vi "参数设置页.vi"() -> ()   [LabVIEW 2016, in "斯坦道氟化物.lvlib"]
uses:
  <vilib>/Plasmionique/MB Master/MB_Master/MB_Master.lvclass
  <vilib>/ptbypt/NI_PtbyPt.lvlib
panel:
  out "连接状态":bool
  in  "标样核查自动补测":bool caption="通讯连接"
  in  "跨度核查自动补测":bool caption="通讯连接"
  in  "零点核查自动补测":bool caption="通讯连接"
  in  "标样核查标液偏差":dbl caption="标样核查标液偏差："
  in  "跨度核查标液偏差":dbl caption="跨度核查标液偏差："
  in  "零点核查标液偏差":dbl caption="零点核查标液偏差："
  out "低量程上限":dbl caption="低量程上限："
  in  "简易流程路径":path=path "data/流程.xml"
  out "数据刷新时间":string
  in  "通讯连接":bool=TRUE
  out "MB table":enum32{"Serial", "TCP"}(tab)
  in  "请选择串口:":refnum<visa-resource-name>
  in  "IP":string="127.0.0.1"
  in  "PORT":string="1001"
  in  "通信方式选择":enum16{"串口", "TCP"}(ring)
  in  "盐度自动补偿：":bool
  out "盐度补偿值":dbl caption="盐度补偿值："
  in  "刷新":bool
  in  "测量模式":T1(ring)
  in  "参数下拉列表":u16(ring)
  in  "量程下拉列表":enum16{"低量程", "高量程"}(ring)
  in  "测试流程路径":path=path "data/流程.xml"
  in  "标样核查量程模式":T2 caption="标样核查："
  in  "加标回收量程模式":T2 caption="加标回收："
  in  "跨度核查量程模式":T2 caption="跨度核查："
  in  "零点核查量程模式":T2 caption="零点核查："
  in  "水样测试量程模式":T2 caption="水样测试："
  out "稀释度":dbl caption="稀释度："
  out "阈值（高->低）":dbl caption="阈值（高->低）："
  out "阈值（低->高）":dbl caption="阈值（低->高）："
  out "量程下限":dbl caption="量程下限："
  out "高量程上限":dbl caption="高量程上限："
  out "检出限":dbl caption="检出限："
  out "曲线截距":dbl caption="曲线截距：" format="%#.6f"
  out "曲线斜率":dbl caption="曲线斜率：" format="%#.6f"
  out "二次多项式系数":dbl caption="二次多项式系数：" format="%#.6f"
  out "消解时长":dbl caption="消解时长："
  out "消解温度":dbl caption="消解温度："
  out "测量精度":u16 caption="测量精度："
  in  "标样核查标液浓度":dbl caption="标样核查标液浓度："
  in  "跨度核查标液浓度":dbl caption="跨度核查标液浓度："
  in  "零点核查标液浓度":dbl caption="零点核查标液浓度："
  in  "跨度值":dbl caption="跨度值："
  # "日质控设置"
  # "关键参数"
  # "连接设置"
  # "mg/L"
  # "mg/L"
  # "mg/L"
  # "mg/L"
  # "±"
  # "%"
  # "%"
  # "流程设置"
  # "自动测试量程设置"
  # "mg/L"
  # "ppt"
  # "mg/L"
  # "mg/L"
  # "mg/L"
  # "mg/L"
  # "mg/L"
  # "min"
  # "℃"
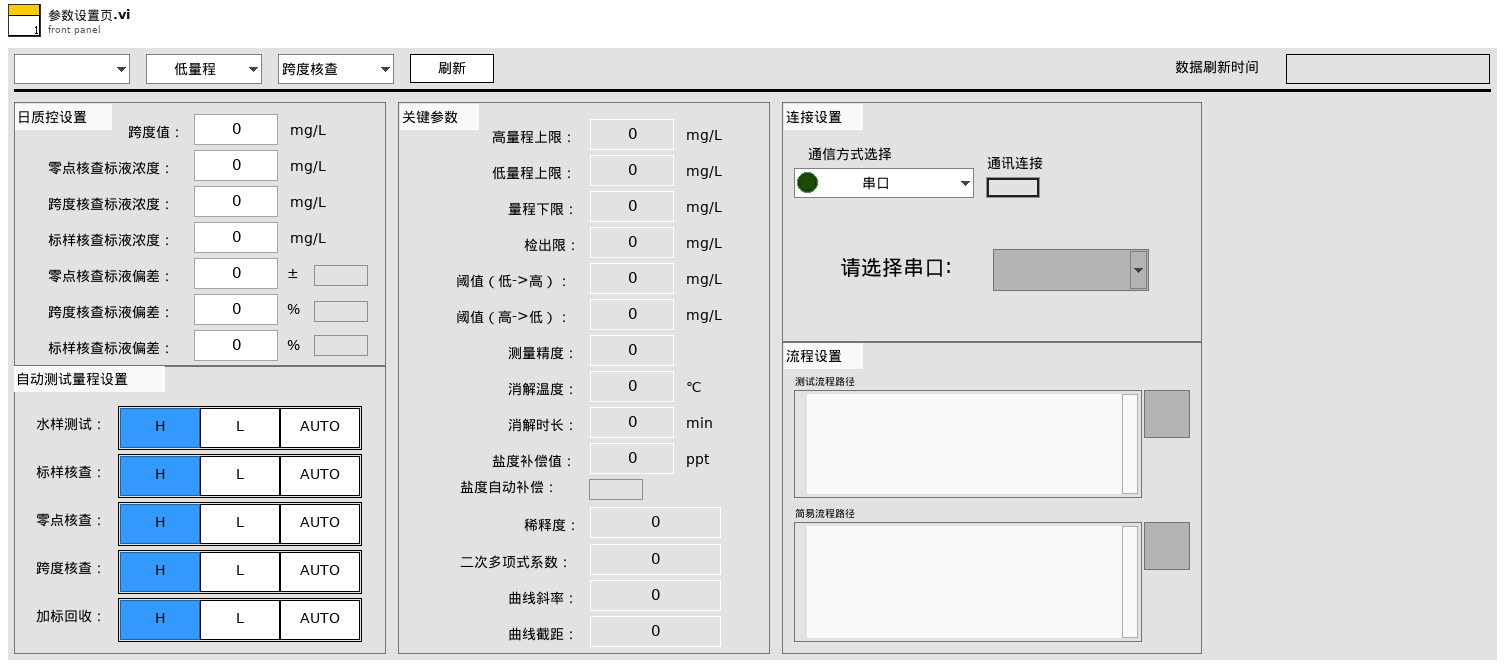
[diagram p1: front panel]
types:
  T1 = enum16{"跨度核查", "水样测量", "零点核查", "标样核查", "加标回收", "快捷测试", "空白校准", "标样校准"}
  T2 = typedef "斯坦道氟化物.lvlib/量程模式.ctl" = enum32{"H", "L", "AUTO"}
  T3 = typedef "LVStringsAndValuesArrayTypeDef_U16.ctl" = cluster{"String":string, "Value":u16}[]
  T4 = cluster{"系统时间":timestamp, "工作状态":u16, "测量模式":enum16{"待机", "连续模式", "周期模式", "定点模式", "受控模式", "手动模式"}, "告警代码":u16, "故障代码":u16, "日志代码":u16, "软件版本":u16, "F0":sgl, "F1":sgl, "F2":sgl, "F3":sgl, "T":sgl, "H":sgl, "id":u16, "flowid":u16, "量程":u16, "总磷控温温度1":sgl, "营养盐控温温度2":sgl, "ADC":sgl}
  T5 = enum8{"Enabled", "Disabled", "Disabled and Grayed Out"}
  T6 = cluster{"测量精度":u16, "检出限":dbl, "上限":dbl, "下限":dbl, "阈值（低->高）":dbl, "阈值（高->低）":dbl, "稀释度":dbl}
  T7 = typedef "操作日志字段定义.ctl" = cluster{"时间":timestamp, "参数":string, "日志信息":string, "流程参数":string}
  T8 = typedef "斯坦道氟化物.lvlib/V3 A版外设参数.ctl" = cluster{"泵类型":u8, "进样速度":u32, "出样速度":u32, "泵阀量":u8, "阀方向":u8, "光谱仪类型":u8, "光谱采样次数":u8, "氙灯次数":u8, "B":u16, "C":u16, "D":u16, "E":u16, "B_COD":u16, "C_COD":u16, "D_COD":u16, "E_COD":u16, "G":u16, "M":u16, "N":u16, "氨氮注射泵控温下限":sgl, "氨氮注射泵控温上限":sgl, "总氮注射泵控温下限":sgl, "总氮注射泵控温上限":sgl, "消解温度下限":sgl, "消解温度上限":sgl, "加热10s限值":sgl, "KP":sgl, "KI":sgl, "KD":sgl, "高温高压阀开阀温度":sgl, "总氮x公式0":u8, "总氮x公式1":sgl, "总氮x公式2":sgl, "总磷浊度稀释系数":sgl, "总磷浊度补偿权重1":sgl, "总磷浊度补偿权重2":sgl, "盐度系数":sgl, "氨氮补偿系数1":sgl, "氨氮补偿系数2":sgl}
  T9 = cluster{"水样测试量程模式":T2, "零点核查量程模式":T2, "跨度核查量程模式":T2, "加标回收量程模式":T2, "标样核查量程模式":T2}
  T10 = cluster{"总磷":dbl, "总氮":dbl, "氨氮":dbl, "磷酸盐":dbl, "硝氮":dbl, "亚硝氮":dbl, "硅酸盐":dbl, "硫化物":dbl, "COD":dbl, "氟化物":dbl, "CODMn":dbl}
  T11 = cluster{"总磷跨度值":dbl, "总磷零点标准液浓度":dbl, "总磷跨度标准液浓度":dbl, "总磷标准液标准浓度":dbl, "总氮跨度值":dbl, "总氮零点标准液浓度":dbl, "总氮跨度标准液浓度":dbl, "总氮标准液标准浓度":dbl, "COD跨度值":dbl, "COD零点标准液浓度":dbl, "COD跨度标准液浓度":dbl, "COD标准液标准浓度":dbl, "氨氮跨度值":dbl, "氨氮零点标准液浓度":dbl, "氨氮跨度标准液浓度":dbl, "氨氮标准液标准浓度":dbl, "磷酸盐跨度值":dbl, "磷酸盐零点标准液浓度":dbl, "磷酸盐跨度标准液浓度":dbl, "磷酸盐标准液标准浓度":dbl, "硝氮跨度值":dbl, "硝氮零点标准液浓度":dbl, "硝氮跨度标准液浓度":dbl, "硝氮标准液标准浓度":dbl, "亚硝氮跨度值":dbl, "亚硝氮零点标准液浓度":dbl, "亚硝氮跨度标准液浓度":dbl, "亚硝氮标准液标准浓度":dbl, "硫化物跨度值":dbl, "硫化物零点标准液浓度":dbl, "硫化物跨度标准液浓度":dbl, "硫化物标准液标准浓度":dbl, "硅酸盐跨度值":dbl, "硅酸盐零点标准液浓度":dbl, "硅酸盐跨度标准液浓度":dbl, "硅酸盐标准液标准浓度":dbl, "总磷零点标准液偏差":dbl, "总磷跨度标准液偏差":dbl, "总磷标准液标准偏差":dbl, "总氮零点标准液偏差":dbl, "总氮跨度标准液偏差":dbl, "总氮标准液标准偏差":dbl, "COD零点标准液偏差":dbl, "COD跨度标准液偏差":dbl, "COD标准液标准偏差":dbl, "氨氮零点标准液偏差":dbl, "氨氮跨度标准液偏差":dbl, "氨氮标准液标准偏差":dbl, "磷酸盐零点标准液偏差":dbl, "磷酸盐跨度标准液偏差":dbl, "磷酸盐标准液标准偏差":dbl, "硝氮零点标准液偏差":dbl, "硝氮跨度标准液偏差":dbl, "硝氮标准液标准偏差":dbl, "亚硝氮零点标准液偏差":dbl, "亚硝氮跨度标准液偏差":dbl, "亚硝氮标准液标准偏差":dbl, "硫化物零点标准液偏差":dbl, "硫化物跨度标准液偏差":dbl, "硫化物标准液标准偏差":dbl, "硅酸盐零点标准液偏差":dbl, "硅酸盐跨度标准液偏差":dbl, "硅酸盐标准液标准偏差":dbl, "氟化物跨度值":dbl, "氟化物零点标准液浓度":dbl, "氟化物跨度标准液浓度":dbl, "氟化物标准液标准浓度":dbl, "氟化物零点标准液偏差":dbl, "氟化物跨度标准液偏差":dbl, "氟化物标准液标准偏差":dbl, "CODMn跨度值":dbl, "CODMn零点标准液浓度":dbl, "CODMn跨度标准液浓度":dbl, "CODMn标准液标准浓度":dbl, "CODMn零点标准液偏差":dbl, "CODMn跨度标准液偏差":dbl, "CODMn标准液标准偏差":dbl}
  T12 = typedef "SingleStepTestV3.lvlib/SingleStepTestV3.lvclass/仪器版本.ctl" = enum16{"A版", "B版", "A1版"}
  T13 = typedef "斯坦道氟化物.lvlib/V3 B版外设参数.ctl" = cluster{"泵类型":u8, "注射泵正常速度":u32, "注射泵慢速":u32, "阀型号":u8, "res":u8, "光谱仪类型":u8, "光谱采样次数":u8, "氙灯次数":u8, "B":u16, "C":u16, "D":u16, "E":u16, "B_COD":u16, "C_COD":u16, "D_COD":u16, "E_COD":u16, "G":u16, "M":u16, "N":u16, "降温下限":sgl, "降温上限":sgl, "恒温温度下限":sgl, "恒温温度上限":sgl, "消解温度下限":sgl, "消解温度上限":sgl, "加热10s限值":sgl, "KP":sgl, "KI":sgl, "KD":sgl, "高温高压阀开阀温度":sgl, "总氮x公式0":u8, "总氮x公式1":sgl, "总氮x公式2":sgl, "总磷浊度稀释系数":sgl, "总磷浊度补偿权重1":sgl, "总磷浊度补偿权重2":sgl, "盐度系数":sgl, "氨氮补偿系数1":sgl, "氨氮补偿系数2":sgl, "缺试剂传感器阈值":u16}
  T14 = typedef "斯坦道氟化物.lvlib/V3 A1版外设参数.ctl" = cluster{"泵类型":u8, "进样速度":u32, "出样速度":u32, "泵阀量":u8, "光谱仪类型":u8, "光谱采样次数":u8, "氙灯次数":u8, "B":u16, "C":u16, "D":u16, "E":u16, "B_COD":u16, "C_COD":u16, "D_COD":u16, "E_COD":u16, "G":u16, "M":u16, "N":u16, "氨氮注射泵控温下限":sgl, "氨氮注射泵控温上限":sgl, "总氮注射泵控温下限":sgl, "总氮注射泵控温上限":sgl, "消解温度下限":sgl, "消解温度上限":sgl, "加热10s限值":sgl, "高温高压阀开阀温度":sgl, "总氮x公式0":u8, "总氮x公式1":sgl, "总氮x公式2":sgl, "总磷浊度稀释系数":sgl, "总磷浊度补偿权重1":sgl, "总磷浊度补偿权重2":sgl, "盐度系数":sgl, "氨氮补偿系数1":sgl, "氨氮补偿系数2":sgl}
  T15 = cluster{"水样测试量程模式":enum16{"H", "L", "AUTO"}, "空白核查量程模式":enum16{"H", "L", "AUTO"}, "跨度核查量程模式":enum16{"H", "L", "AUTO"}, "加标回收量程模式":enum16{"H", "L", "AUTO"}, "标样核查量程模式":enum16{"H", "L", "AUTO"}}
  T16 = cluster{"水样测试量程模式":u16, "空白核查量程模式":u16, "跨度核查量程模式":u16, "加标回收量程模式":u16, "标样核查量程模式":u16}
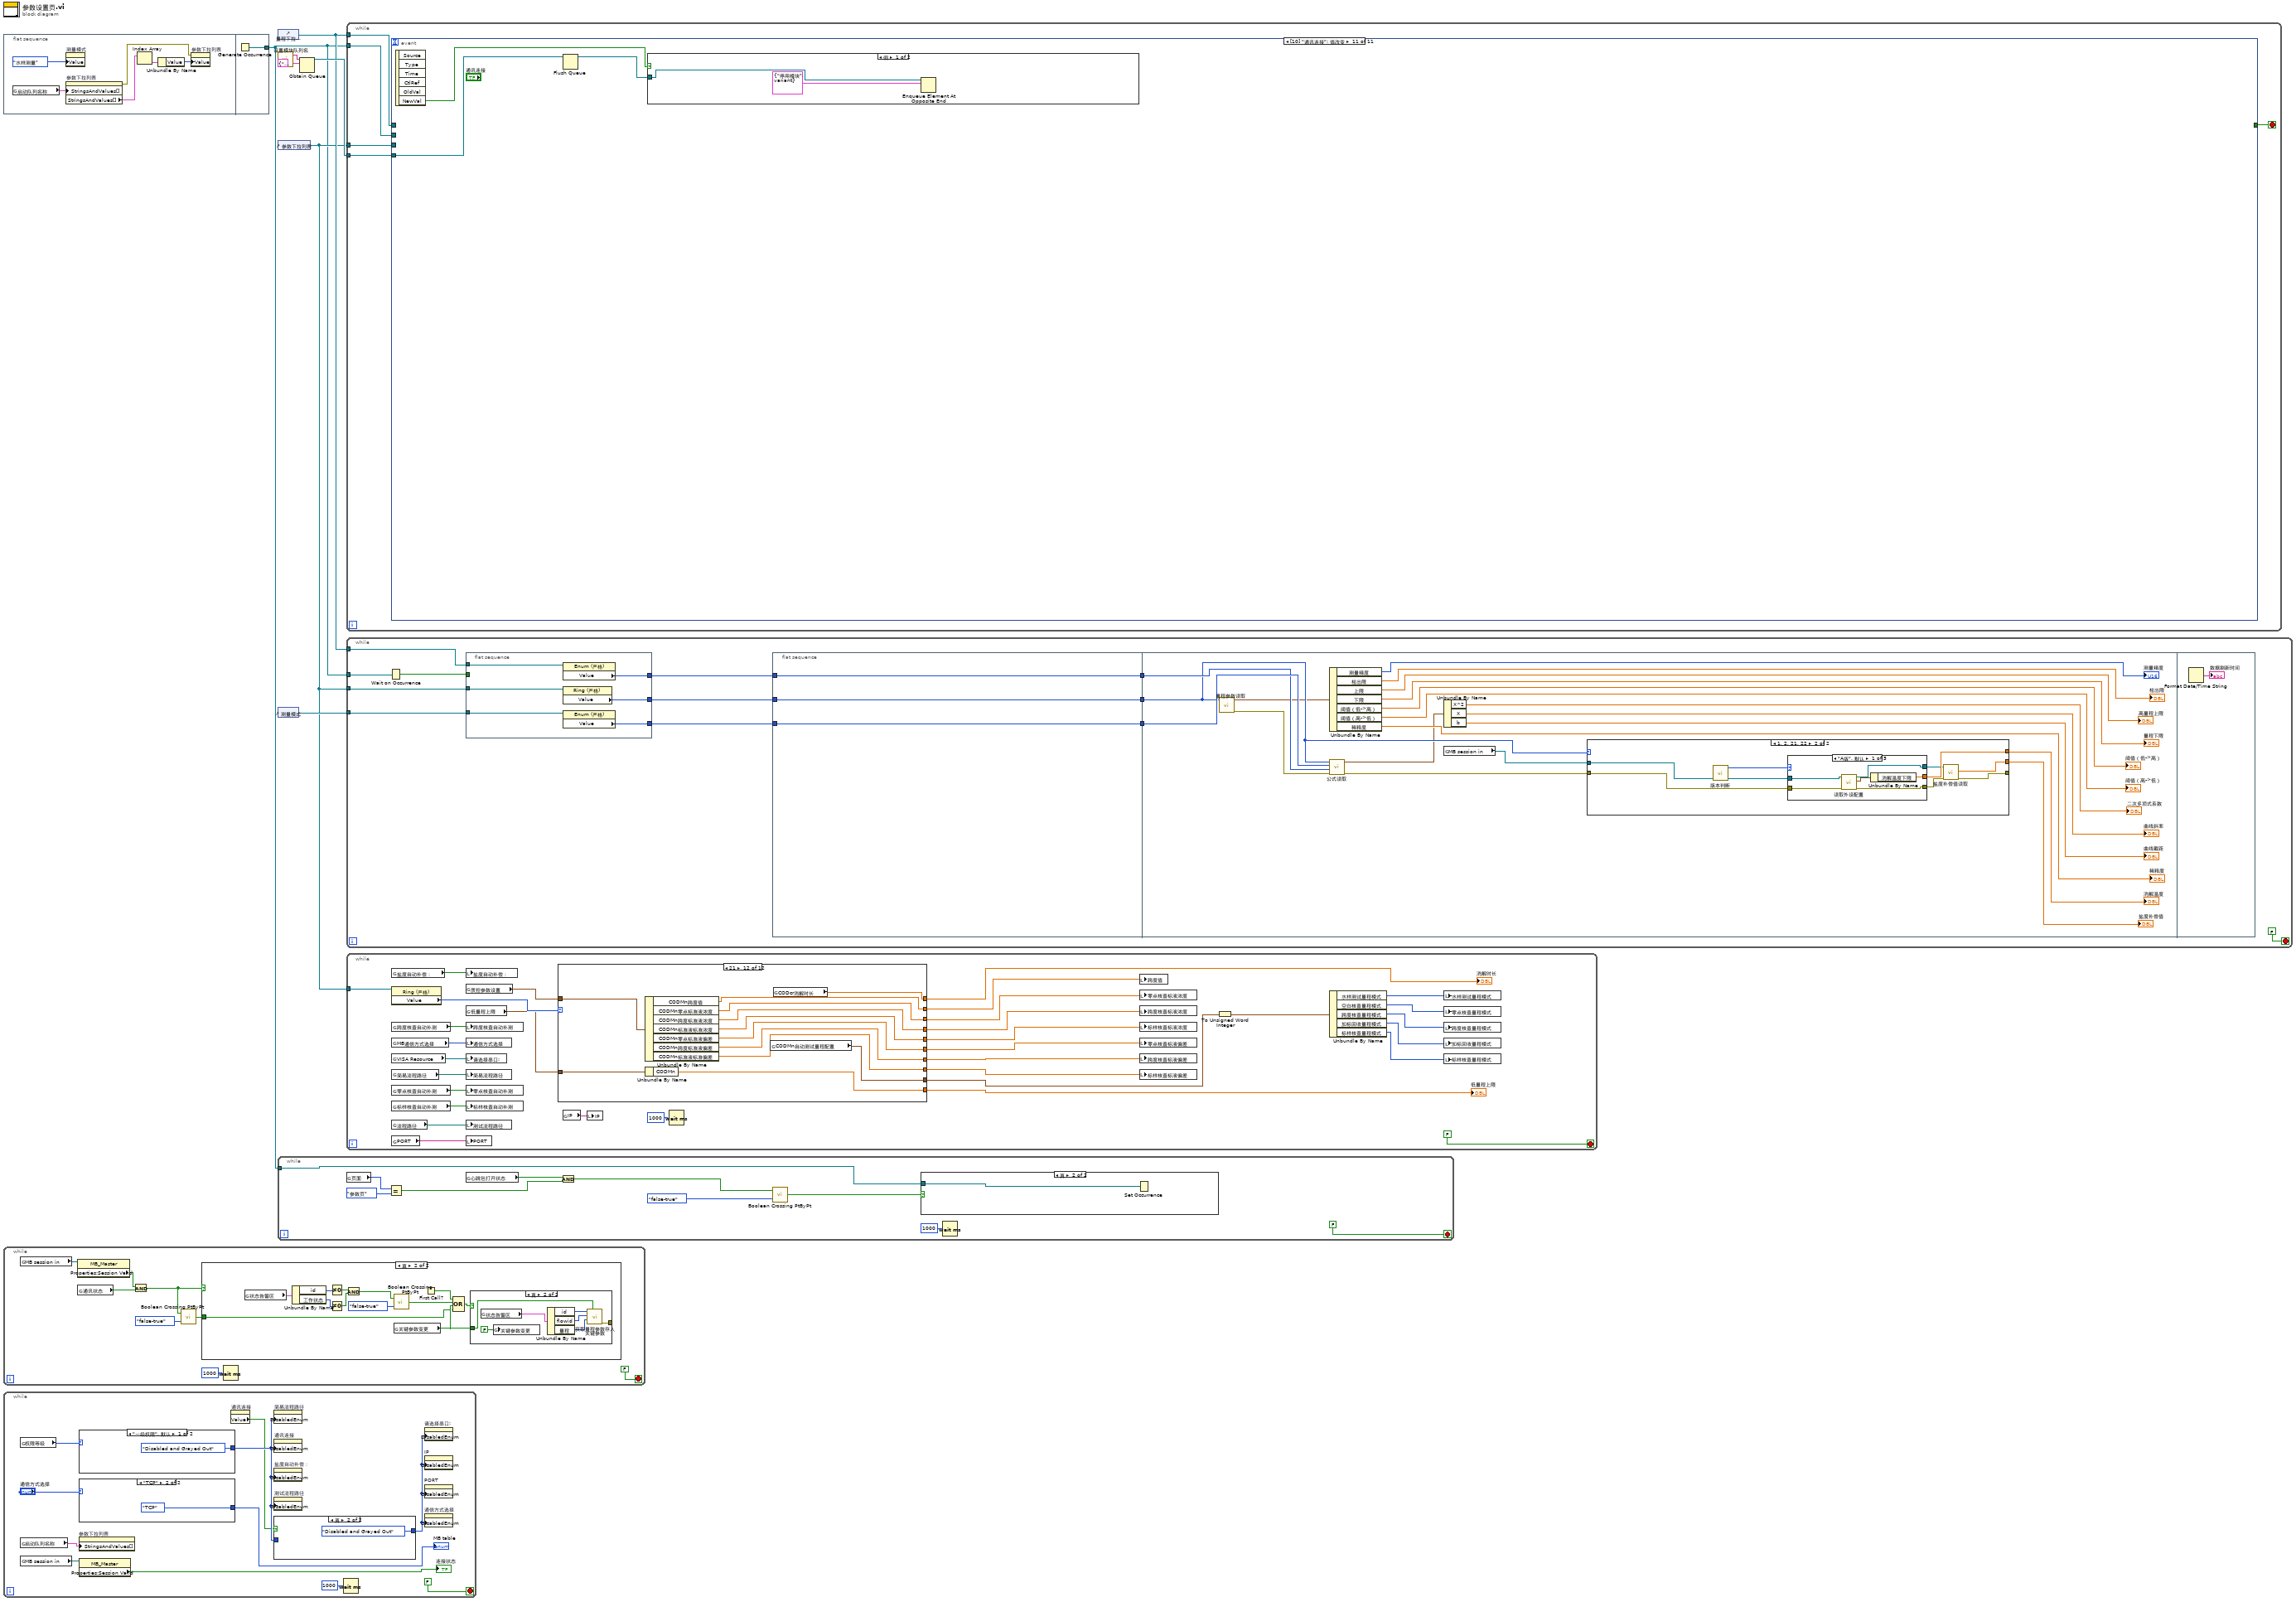
[diagram p0: block diagram]
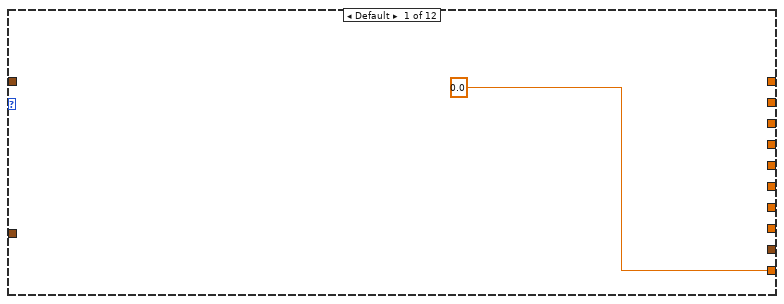
[diagram p5: hidden frame]
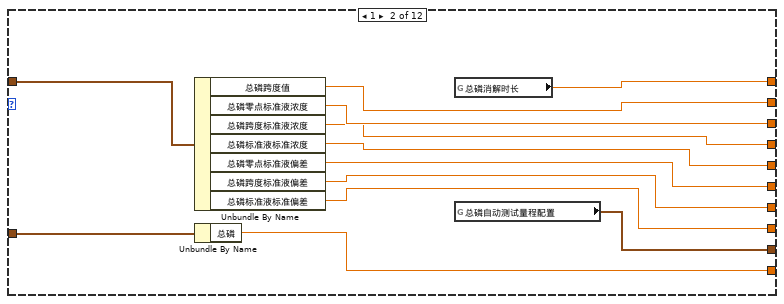
[diagram p6: hidden frame]
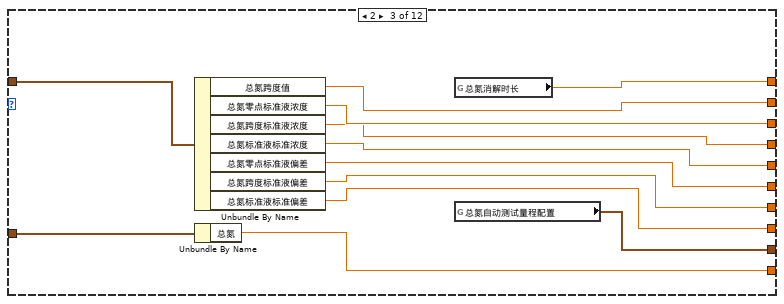
[diagram p7: hidden frame]
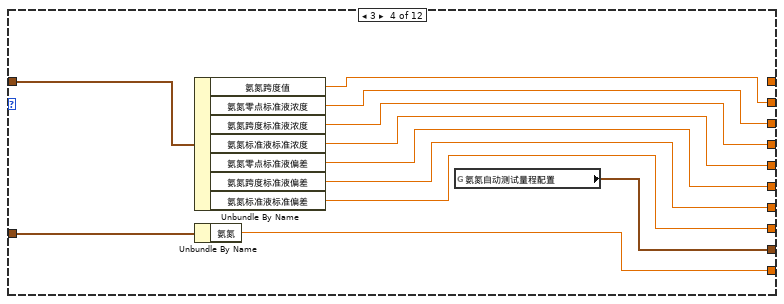
[diagram p8: hidden frame]
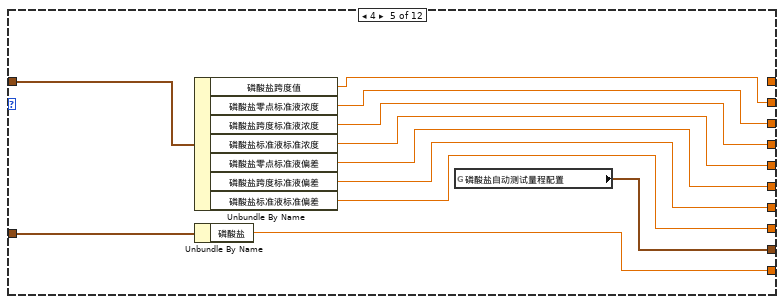
[diagram p9: hidden frame]
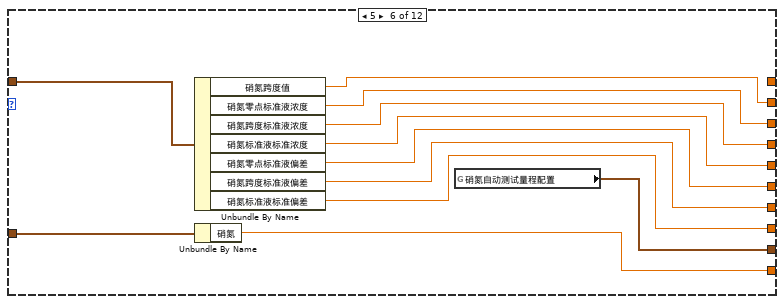
[diagram p10: hidden frame]
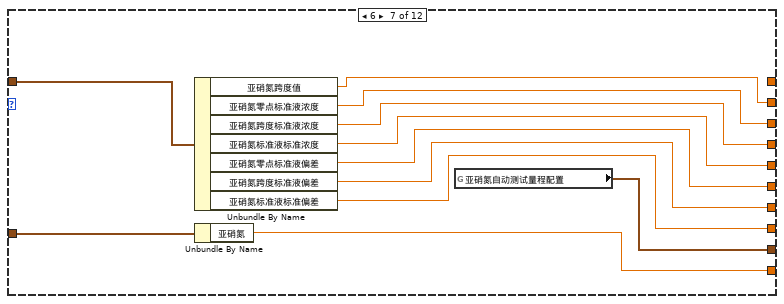
[diagram p11: hidden frame]
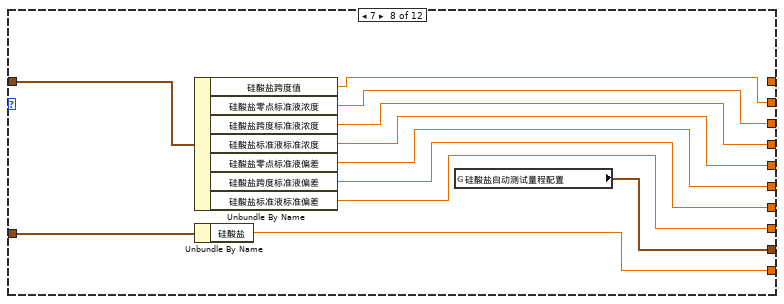
[diagram p12: hidden frame]
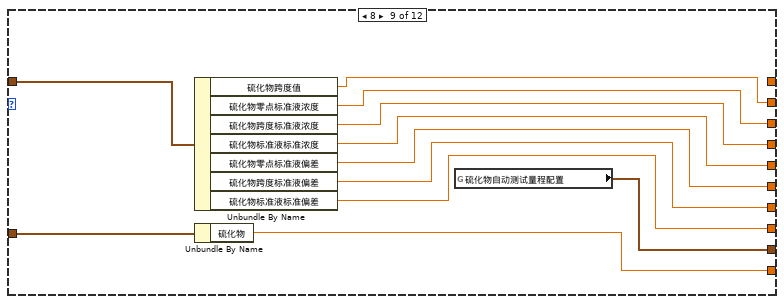
[diagram p13: hidden frame]
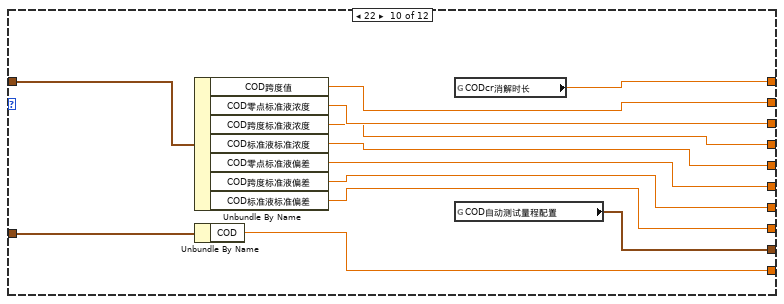
[diagram p14: hidden frame]
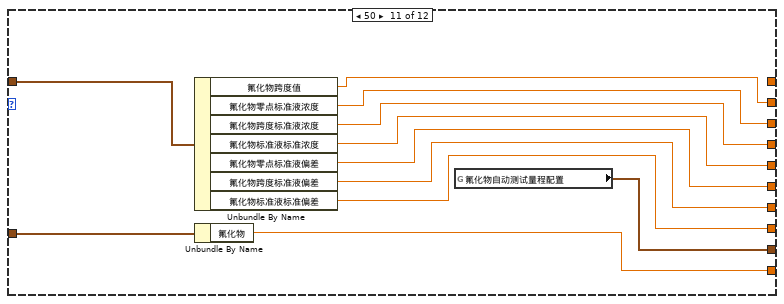
[diagram p15: hidden frame]
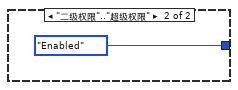
[diagram p16: hidden frame]
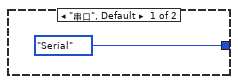
[diagram p17: hidden frame]
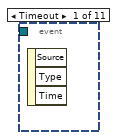
[diagram p19: hidden frame]
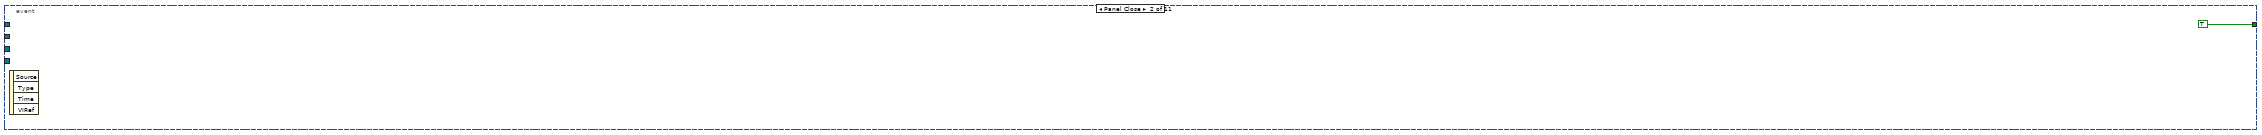
[diagram p20: hidden frame]
diagram:
  n1 = flat-sequence {
    tunnel: [w14] -> w1
    frame #0 {
      n2 = global read "model config var.vi" "启动队列名称"() -> (w9:cluster{"String":string, "Value":u16}[])
      n3 = property on="测量模式" class="Enum (严格)"("Value"=T1."水样测量" ("测量模式")) -> ()  [unwired: 2 in, 2 out]
      n4 = property on="参数下拉列表" class="Ring (严格)"("StringsAndValues[]"=w9) -> (error out=w12:errorcluster, "StringsAndValues[]"=w10:T3)  [unwired: 2 in, 1 out]
      n5 = Index Array(array=w10) -> (element=w11:cluster{"String":string, "Value":u16})  [unwired: 1 in]
      n6 = Unbundle By Name(w11) -> ("Value"=w13:u16)
      n7 = property on="参数下拉列表" class="Ring (严格)"(error in=w12, "Value"=w13) -> ()  [unwired: 1 in, 2 out]
    }
    frame #1 {
      n8 = Generate Occurrence() -> (w14:refnum<k4>)
    }
  }
  n9 = while {
    stop <- FALSE stop-if-true
    n10 = global read "VAR总磷总氮全局变量.vi" "MB session in"() -> (w19:refnum<class "MB_Master.lvclass">)
    n11 = property class="MB_Master"(reference=w19) -> ("Properties:Session Valid"=w18:bool)  [unwired: 1 in, 2 out]
    n12 = global read "VAR总磷总氮全局变量.vi" "通讯状态"() -> (w21:bool)
    n13 = And(x=w18, y=w21) -> (x .and. y?=w16:bool)
    n14 = call <vilib>:"Boolean Crossing PtByPt.vi"("direction"=enum16{"either", "false-true", "true-false"}."false-true", "input"=w16) -> ("crossing"=w15:bool)  [unwired: 1 in]
    n15 = case shown="真" w16 {
      tunnel: w15 -> [_ w24]
      frame False {
      }
      frame True {
        n16 = global read "VAR总磷总氮全局变量.vi" "状态告警区"() -> (w34:T4)
        n17 = Unbundle By Name(w34) -> ("id"=w28:u16, "工作状态"=w33:u16)
        n18 = Not Equal To 0?(x=w28) -> (x != 0?=w29:bool)
        n19 = Not Equal To 0?(x=w33) -> (x != 0?=w30:bool)
        n20 = And(x=w29, y=w30) -> (x .and. y?=w31:bool)
        n21 = call <vilib>:"Boolean Crossing PtByPt.vi"("direction"=enum16{"either", "false-true", "true-false"}."false-true", "input"=w31) -> ("crossing"=w27:bool)  [unwired: 1 in]
        n22 = global read "VAR总磷总氮全局变量.vi" "关键参数变更"() -> (w25:bool)
        n23 = First Call?() -> (First Call?: T/F=w23:bool)
        n24 = Compound Arithmetic op=OR ("复合运算")(w23, w27, w25, w24) -> (w26:bool)
        n25 = case shown="真" w26 {
          tunnel: [_ w41] -> _
          tunnel: w25 -> [_ w36]
          frame False {
          }
          frame True {
            n26 = global read "VAR总磷总氮全局变量.vi" "状态告警区"() -> (w40:T4)
            n27 = global write "VAR总磷总氮全局变量.vi" "关键参数变更"(FALSE ("关键参数变更")) -> ()
            n28 = Unbundle By Name(w40) -> ("id"=w39:u16, "flowid"=w38:u16, "量程"=w37:u16)
            n29 = call "获取量程参数存入关键参数.vi"("关键参数变更"=w36, "量程"=w37, "flowid"=w38, "id"=w39) -> ("error out"=w41:errorcluster)  [unwired: 7 in]
          }
        }
      }
    }
    n30 = Wait (ms)(milliseconds to wait=u32 1000 ("等待时间（毫秒）")) -> ()  [unwired: 1 out]
  }
  n31 = while {
    stop <- FALSE stop-if-true
    n32 = global read "VAR总磷总氮全局变量.vi" "权限等级"() -> (w46:enum16{"一级权限", "二级权限", "三级权限", "超级权限"})
    n33 = global read "model config var.vi" "启动队列名称"() -> (w44:cluster{"String":string, "Value":u16}[])
    n34 = global read "VAR总磷总氮全局变量.vi" "MB session in"() -> (w51:refnum<class "MB_Master.lvclass">)
    n35 = case shown="\"一级权限\", 默认" w46 {
      tunnel: [T5."Disabled and Grayed Out" ("禁用") T5."Enabled" ("禁用")] -> w45
      frame "一级权限", Default {
      }
      frame "二级权限".."超级权限" {
      }
    }
    n36 = case shown="\"TCP\"" "通信方式选择" {
      tunnel: [enum32{"Serial", "TCP"}."Serial" ("MB table") enum32{"Serial", "TCP"}."TCP" ("MB table")] -> w48
      frame "串口", Default {
      }
      frame "TCP" {
      }
    }
    "MB table" <- w48
    n37 = property on="参数下拉列表" class="Ring (严格)"("StringsAndValues[]"=w44) -> ()  [unwired: 2 in, 2 out]
    n38 = property class="MB_Master"(reference=w51) -> ("Properties:Session Valid"=→"连接状态":bool)  [unwired: 1 in, 2 out]
    n39 = property on="通讯连接" class="Bool (严格)"() -> ("Value"=w42:bool)  [unwired: 2 in, 2 out]
    n40 = property on="简易流程路径" class="Path"("DisabledEnum"=w45) -> ()  [unwired: 2 in, 2 out]
    n41 = property on="通讯连接" class="Bool (严格)"("DisabledEnum"=w45) -> ()  [unwired: 2 in, 2 out]
    n42 = property on="盐度自动补偿：" class="Bool (严格)"("DisabledEnum"=w45) -> ()  [unwired: 2 in, 2 out]
    n43 = property on="测试流程路径" class="Path"("DisabledEnum"=w45) -> ()  [unwired: 2 in, 2 out]
    n44 = case shown="真" w42 {
      tunnel: [w57 T5."Disabled and Grayed Out" ("禁用")] -> w49
      tunnel: w45 -> [w57 _]
      frame False {
      }
      frame True {
      }
    }
    n45 = Wait (ms)(milliseconds to wait=u32 1000 ("等待时间（毫秒）")) -> ()  [unwired: 1 out]
    n46 = property on="请选择串口:" class="VISAName"("DisabledEnum"=w49) -> ()  [unwired: 2 in, 2 out]
    n47 = property on="IP" class="Str"("DisabledEnum"=w49) -> ()  [unwired: 2 in, 2 out]
    n48 = property on="PORT" class="Str"("DisabledEnum"=w49) -> ()  [unwired: 2 in, 2 out]
    n49 = property on="通信方式选择" class="Enum (严格)"("DisabledEnum"=w49) -> ()  [unwired: 2 in, 2 out]
  }
  n50 = control-ref of="量程下拉列表"() -> (w3:refnum<vi>)
  n51 = call "设置模块队列名.vi"() -> ("Msg"=w6:string)  [unwired: 5 in]
  n52 = control-ref of="参数下拉列表"() -> (w2:refnum<vi>)
  n53 = control-ref of="测量模式"() -> (w4:refnum<vi>)
  n54 = while {
    tunnel: w1 -> [w65]
    stop <- FALSE stop-if-true
    n55 = global read "VAR总磷总氮全局变量.vi" "页面"() -> (w67:enum16{"主页", "参数页", "校准页"})
    n56 = Equal?(x=w67, y=enum16{"主页", "参数页", "校准页"}."参数页" ("页面")) -> (x = y?=w66:bool)
    n57 = global read "VAR总磷总氮全局变量.vi" "心跳包打开状态"() -> (w61:bool)
    n58 = And(x=w61, y=w66) -> (x .and. y?=w62:bool)
    n59 = call <vilib>:"Boolean Crossing PtByPt.vi"("direction"=enum16{"either", "false-true", "true-false"}."false-true", "input"=w62) -> ("crossing"=w60:bool)  [unwired: 1 in]
    n60 = case shown="真" w60 {
      tunnel: w65 -> [_ w69]
      frame False {
      }
      frame True {
        n61 = Set Occurrence(w69) -> ()
      }
    }
    n62 = Wait (ms)(milliseconds to wait=u32 1000 ("等待时间（毫秒）")) -> ()  [unwired: 1 out]
  }
  n63 = Obtain Queue(name (unnamed)=w6, element data type=cluster{"命令":string, "data":variant} {"命令"="", "data"=variant}) -> (queue out=w5:refnum<queue>)  [unwired: 3 in, 2 out]
  n64 = while {
    tunnel: w1 -> [w73]
    tunnel: w2 -> [w72]
    tunnel: w5 -> [w71]
    tunnel: w3 -> [w70]
    stop <- w74 stop-if-true
    n65 = event shown="[10] \"通讯连接\": 值改变" {
      selector: _ -> [_ _ _ _ _ _ _ _ _ _ _]
      dyn-events: _ -> [_ _ _ _ _ _ _ _ _ _ _]
      timeout: _ -> [_ _ _ _ _ _ _ _ _ _ _]
      tunnel: [_ TRUE _ _ _ _ _ _ _ _ _] -> w74
      tunnel: w73 -> [_ _ w76 _ _ _ _ _ _ w129 _]
      tunnel: w72 -> [_ _ _ _ w95 _ _ _ _ w131 _]
      tunnel: w71 -> [_ _ _ _ _ _ _ _ _ _ w319]
      tunnel: w70 -> [_ _ _ _ _ _ _ _ _ _ _]
      event Timeout {
        n66 = event-data() -> ()  [unwired: 1 in, 3 out]
      }
      event Panel Close {
        n67 = event-data() -> ()  [unwired: 1 in, 4 out]
      }
      event "参数下拉列表", "量程下拉列表", "测量模式", "刷新": Value Change {
        n68 = event-data() -> ()  [unwired: 1 in, 6 out]
        n69 = Set Occurrence(w76) -> ()
      }
      event "跨度值", "零点核查标液浓度", "跨度核查标液浓度", "标样核查标液浓度", "消解温度", "消解时长", "检出限", "高量程上限", "量程下限", "阈值（低->高）", "阈值（高->低）", "稀释度", "低量程上限", "零点核查标液偏差", "跨度核查标液偏差", "标样核查标液偏差": Mouse Down {
        n70 = event-data() -> ("CtlRef"=w78:refnum<vi>)  [unwired: 1 in, 5 out]
        n71 = global read "VAR总磷总氮全局变量.vi" "权限等级"() -> (w77:enum16{"一级权限", "二级权限", "三级权限", "超级权限"})
        n72 = case shown="\"二级权限\"..\"超级权限\"" w77 {
          tunnel: w78 -> [_ w82]
          frame "一级权限", Default {
          }
          frame "二级权限".."超级权限" {
            n73 = property class="DigNum (严格)"(reference=w82) -> (reference out=w80:refnum<vi>, "Value"=w81:dbl)  [unwired: 1 in, 1 out]
            n74 = call "数字键盘.vi"("OldNumber"=w81) -> ("NewNumber"=w79:dbl)
            n75 = property class="DigNum (严格)"(reference=w80, "Val(Sgnl)"=w79) -> ()  [unwired: 1 in, 2 out]
          }
        }
      }
      event "测量精度", "检出限", "高量程上限", "量程下限", "阈值（低->高）", "阈值（高->低）", "稀释度": Value Change {
        n76 = event-data() -> ()  [unwired: 1 in, 6 out]
        n77 = local read "测量精度"() -> (w85:u16)
        n78 = local read "检出限"() -> (w89:dbl)
        n79 = local read "高量程上限"() -> (w91:dbl)
        n80 = local read "量程下限"() -> (w90:dbl)
        n81 = local read "阈值（低->高）"() -> (w88:dbl)
        n82 = local read "阈值（高->低）"() -> (w87:dbl)
        n83 = local read "稀释度"() -> (w86:dbl)
        n84 = property class="Ring (严格)"(reference=w95) -> ("Value"=w94:u16)  [unwired: 1 in, 2 out]
        n85 = Bundle By Name(cluster=T6 {"测量精度"=0, "检出限"=0.0, "上限"=0.0, "下限"=0.0, "阈值（低->高）"=0.0, "阈值（高->低）"=0.0, "稀释度"=0.0} ("量程参数写入"), "测量精度"=w85, "检出限"=w89, "上限"=w91, "下限"=w90, "阈值（低->高）"=w88, "阈值（高->低）"=w87, "稀释度"=w86) -> (w92:T6)
        n86 = call "量程参数写入.vi"("量程参数写入"=w92, "测量参数"=w94) -> ("error out"=w83:errorcluster)  [unwired: 8 in]
        n87 = case shown="无错误" w83 {
          tunnel: ["写入成功" "写入失败"] -> w84
          frame No Error {
            n88 = Get Date/Time In Seconds() -> (seconds since 1Jan1904=w98:timestamp)
            n89 = property on="参数下拉列表" class="Ring (严格)"() -> ("RingText.Text"=w96:string)  [unwired: 2 in, 2 out]
            n90 = Bundle By Name(cluster=T7 {"时间"=timestamp(0 s since 1904-01-01), "参数"="", "日志信息"="", "流程参数"=""} ("data in"), "时间"=w98, "参数"=w96, "日志信息"="关键参数变更") -> (w99:T7)
            n91 = call "总磷总氮操作日志.vi"("data in"=w99) -> ()  [unwired: 10 in, 1 out]
            n92 = global write "VAR总磷总氮全局变量.vi" "关键参数变更"(TRUE ("关键参数变更")) -> ()
          }
          frame Error {
          }
        }
        n93 = One Button Dialog(message=w84) -> ()  [unwired: 1 in, 1 out]
      }
      event "消解温度": Value Change {
        n94 = event-data() -> ("NewVal"=w106:dbl)  [unwired: 1 in, 5 out]
        n95 = global read "VAR总磷总氮全局变量.vi" "MB session in"() -> (w107:refnum<class "MB_Master.lvclass">)
        n96 = call "读取外设配置.vi"("MB session in"=w107) -> ("error out"=w110:errorcluster, "外设配置"=w109:T8)  [unwired: 8 in, 1 out]
        n97 = Bundle By Name(cluster=w109, "消解温度下限"=w106) -> (w108:T8)
        n98 = call "写入外设配置.vi"("error in (no error)"=w110, "外设配置"=w108, "MB session in"=w107) -> ("error out"=w105:errorcluster)  [unwired: 7 in, 1 out]
        n99 = case shown="错误" w105 {
          tunnel: ["写入成功" "写入失败"] -> w104
          frame No Error {
          }
          frame Error {
          }
        }
        n100 = One Button Dialog(message=w104) -> ()  [unwired: 1 in, 1 out]
      }
      event "测量精度": Mouse Down {
        n101 = event-data() -> ("CtlRef"=w114:refnum<vi>)  [unwired: 1 in, 7 out]
        n102 = global read "VAR总磷总氮全局变量.vi" "权限等级"() -> (w113:enum16{"一级权限", "二级权限", "三级权限", "超级权限"})
        n103 = case shown="\"二级权限\"..\"超级权限\"" w113 {
          tunnel: w114 -> [_ w118]
          frame "一级权限", Default {
          }
          frame "二级权限".."超级权限" {
            n104 = property class="DigNum (严格)"(reference=w118) -> (reference out=w116:refnum<vi>, "Value"=w117:u16)  [unwired: 1 in, 1 out]
            n105 = call "数字键盘.vi"("OldNumber"=w117) -> ("NewNumber"=w115:dbl)
            n106 = property class="DigNum (严格)"(reference=w116, "Val(Sgnl)"=w115) -> ()  [unwired: 1 in, 2 out]
          }
        }
      }
      event "盐度补偿值": Mouse Down {
        n107 = event-data() -> ("CtlRef"=w120:refnum<vi>)  [unwired: 1 in, 3 out]
        n108 = global read "VAR总磷总氮全局变量.vi" "权限等级"() -> (w119:enum16{"一级权限", "二级权限", "三级权限", "超级权限"})
        n109 = case shown="\"二级权限\"..\"超级权限\"" w119 {
          tunnel: w120 -> [_ w122]
          frame "一级权限", Default {
          }
          frame "二级权限".."超级权限" {
            n110 = case shown="假" "盐度自动补偿：" {
              tunnel: w122 -> [w126 _]
              frame False {
                n111 = property class="DigNum (严格)"(reference=w126) -> (reference out=w124:refnum<vi>, "Value"=w125:dbl)  [unwired: 1 in, 1 out]
                n112 = call "数字键盘.vi"("OldNumber"=w125) -> ("NewNumber"=w123:dbl)
                n113 = property class="DigNum (严格)"(reference=w124, "Val(Sgnl)"=w123) -> ()  [unwired: 1 in, 2 out]
              }
              frame True {
              }
            }
          }
        }
      }
      event "盐度补偿值": Value Change {
        n114 = event-data() -> ("NewVal"=w127:dbl)  [unwired: 1 in, 5 out]
        n115 = global read "VAR总磷总氮全局变量.vi" "MB session in"() -> (w128:refnum<class "MB_Master.lvclass">)
        n116 = call "盐度补偿值写入.vi"("盐度补偿值"=w127, "MB session in"=w128) -> ()  [unwired: 8 in, 2 out]
      }
      event "跨度值", "零点核查标液浓度", "跨度核查标液浓度", "标样核查标液浓度", "消解时长", "测试流程路径", "盐度自动补偿：", "IP", "PORT", "请选择串口:", "通信方式选择", "简易流程路径", "低量程上限", "零点核查标液偏差", "跨度核查标液偏差", "标样核查标液偏差", "零点核查自动补测", "跨度核查自动补测", "标样核查自动补测": Value Change {
        n117 = event-data() -> ()  [unwired: 1 in, 6 out]
        n118 = global read "VAR总磷总氮全局变量.vi" "权限等级"() -> (w130:enum16{"一级权限", "二级权限", "三级权限", "超级权限"})
        n119 = case shown="\"二级权限\"..\"超级权限\"" w130 {
          tunnel: w131 -> [_ w133]
          tunnel: w129 -> [w132 _]
          frame "一级权限", Default {
            n120 = Set Occurrence(w132) -> ()
          }
          frame "二级权限".."超级权限" {
            n121 = flat-sequence {
              tunnel: w133 -> [w163]
              frame #0 {
                n122 = local read "通信方式选择"() -> (w145:enum16{"串口", "TCP"})
                n123 = property class="Ring (严格)"(reference=w163) -> ("Value"=w162:u16)  [unwired: 1 in, 2 out]
                n124 = local read "盐度自动补偿："() -> (w149:bool)
                n125 = global write "总磷总氮断电保存全局变量.vi" "MB通信方式选择"(w145) -> ()
                n126 = Bundle("水样测试量程模式"="水样测试量程模式", "零点核查量程模式"="零点核查量程模式", "跨度核查量程模式"="跨度核查量程模式", "加标回收量程模式"="加标回收量程模式", "标样核查量程模式"="标样核查量程模式") -> (w151:T9)  [unwired: 1 in]
                n127 = global write "总磷总氮断电保存全局变量.vi" "简易流程路径"("简易流程路径") -> ()
                n128 = global write "总磷总氮断电保存全局变量.vi" "IP"("IP") -> ()
                n129 = global write "总磷总氮断电保存全局变量.vi" "盐度自动补偿："(w149) -> ()
                n130 = global write "总磷总氮断电保存全局变量.vi" "流程路径"("测试流程路径") -> ()
                n131 = global write "总磷总氮断电保存全局变量.vi" "标样核查自动补测"("标样核查自动补测") -> ()
                n132 = global write "总磷总氮断电保存全局变量.vi" "PORT"("PORT") -> ()
                n133 = global write "总磷总氮断电保存全局变量.vi" "跨度核查自动补测"("跨度核查自动补测") -> ()
                n134 = global write "总磷总氮断电保存全局变量.vi" "VISA Resource"("请选择串口:") -> ()
                n135 = global write "总磷总氮断电保存全局变量.vi" "零点核查自动补测"("零点核查自动补测") -> ()
                n136 = To Unsigned Word Integer(number=w151) -> (unsigned 16bit integer=w150:cluster{u16, u16, u16, u16, u16})
                n137 = global read "总磷总氮断电保存全局变量.vi" "低量程上限"() -> (w142:T10)
                n138 = property on="低量程上限" class="DigNum (严格)"() -> ("Value"=w140:dbl)  [unwired: 2 in, 2 out]
                n139 = global read "总磷总氮断电保存全局变量.vi" "质控参数设置"() -> (w157:T11)
                n140 = local read "消解时长"() -> (w144:dbl)
                n141 = case shown="21" w162 {
                  tunnel: "跨度值" -> [_ w177 w191 w204 w217 w230 w243 w256 w269 w283 w297 w310]
                  tunnel: "标样核查标液浓度" -> [_ w174 w188 w201 w214 w227 w240 w253 w266 w280 w294 w307]
                  tunnel: "跨度核查标液浓度" -> [_ w175 w189 w202 w215 w228 w241 w254 w267 w281 w295 w308]
                  tunnel: "零点核查标液浓度" -> [_ w176 w190 w203 w216 w229 w242 w255 w268 w282 w296 w309]
                  tunnel: w157 -> [_ w179 w193 w206 w219 w232 w245 w258 w271 w285 w299 w312]
                  tunnel: w150 -> [_ w173 w187 w200 w213 w226 w239 w252 w265 w278 w292 w306]
                  tunnel: w144 -> [_ w172 w186 _ _ _ _ _ _ w279 w293 _]
                  tunnel: w142 -> [w165 w170 w185 w199 w212 w225 w238 w251 w264 w277 w291 w305]
                  tunnel: [w165 w169 w183 w198 w211 w224 w237 w250 w263 w276 w290 w304] -> w141
                  tunnel: w140 -> [_ w171 w184 w197 w210 w223 w236 w249 w262 w275 w289 w303]
                  tunnel: "标样核查标液偏差" -> [_ w168 w180 w194 w207 w222 w233 w246 w259 w272 w286 w300]
                  tunnel: "跨度核查标液偏差" -> [_ w167 w181 w195 w208 w221 w234 w247 w260 w273 w287 w301]
                  tunnel: "零点核查标液偏差" -> [_ w166 w182 w196 w209 w220 w235 w248 w261 w274 w288 w302]
                  frame 0, Default {
                  }
                  frame 1 {
                    n142 = global write "总磷总氮断电保存全局变量.vi" "总磷自动测试量程配置"(w173) -> ()
                    n143 = global write "总磷总氮断电保存全局变量.vi" "总磷消解时长"(w172) -> ()
                    n144 = Bundle By Name(cluster=w170, "总磷"=w171) -> (w169:T10)
                    n145 = Bundle By Name(cluster=w179, "总磷跨度值"=w177, "总磷零点标准液浓度"=w176, "总磷跨度标准液浓度"=w175, "总磷标准液标准浓度"=w174, "总磷零点标准液偏差"=w166, "总磷跨度标准液偏差"=w167, "总磷标准液标准偏差"=w168) -> (w178:T11)
                    n146 = global write "总磷总氮断电保存全局变量.vi" "质控参数设置"(w178) -> ()
                  }
                  frame 2 {
                    n147 = global write "总磷总氮断电保存全局变量.vi" "总氮自动测试量程配置"(w187) -> ()
                    n148 = global write "总磷总氮断电保存全局变量.vi" "总氮消解时长"(w186) -> ()
                    n149 = Bundle By Name(cluster=w185, "总氮"=w184) -> (w183:T10)
                    n150 = Bundle By Name(cluster=w193, "总氮跨度值"=w191, "总氮零点标准液浓度"=w190, "总氮跨度标准液浓度"=w189, "总氮标准液标准浓度"=w188, "总氮零点标准液偏差"=w182, "总氮跨度标准液偏差"=w181, "总氮标准液标准偏差"=w180) -> (w192:T11)
                    n151 = global write "总磷总氮断电保存全局变量.vi" "质控参数设置"(w192) -> ()
                  }
                  frame 3 {
                    n152 = global write "总磷总氮断电保存全局变量.vi" "氨氮自动测试量程配置"(w200) -> ()
                    n153 = Bundle By Name(cluster=w199, "氨氮"=w197) -> (w198:T10)
                    n154 = Bundle By Name(cluster=w206, "氨氮跨度值"=w204, "氨氮零点标准液浓度"=w203, "氨氮跨度标准液浓度"=w202, "氨氮标准液标准浓度"=w201, "氨氮零点标准液偏差"=w196, "氨氮跨度标准液偏差"=w195, "氨氮标准液标准偏差"=w194) -> (w205:T11)
                    n155 = global write "总磷总氮断电保存全局变量.vi" "质控参数设置"(w205) -> ()
                  }
                  frame 4 {
                    n156 = global write "总磷总氮断电保存全局变量.vi" "磷酸盐自动测试量程配置"(w213) -> ()
                    n157 = Bundle By Name(cluster=w212, "磷酸盐"=w210) -> (w211:T10)
                    n158 = Bundle By Name(cluster=w219, "磷酸盐跨度值"=w217, "磷酸盐零点标准液浓度"=w216, "磷酸盐跨度标准液浓度"=w215, "磷酸盐标准液标准浓度"=w214, "磷酸盐零点标准液偏差"=w209, "磷酸盐跨度标准液偏差"=w208, "磷酸盐标准液标准偏差"=w207) -> (w218:T11)
                    n159 = global write "总磷总氮断电保存全局变量.vi" "质控参数设置"(w218) -> ()
                  }
                  frame 5 {
                    n160 = global write "总磷总氮断电保存全局变量.vi" "硝氮自动测试量程配置"(w226) -> ()
                    n161 = Bundle By Name(cluster=w225, "硝氮"=w223) -> (w224:T10)
                    n162 = Bundle By Name(cluster=w232, "硝氮跨度值"=w230, "硝氮零点标准液浓度"=w229, "硝氮跨度标准液浓度"=w228, "硝氮标准液标准浓度"=w227, "硝氮零点标准液偏差"=w220, "硝氮跨度标准液偏差"=w221, "硝氮标准液标准偏差"=w222) -> (w231:T11)
                    n163 = global write "总磷总氮断电保存全局变量.vi" "质控参数设置"(w231) -> ()
                  }
                  frame 6 {
                    n164 = global write "总磷总氮断电保存全局变量.vi" "亚硝氮自动测试量程配置"(w239) -> ()
                    n165 = Bundle By Name(cluster=w238, "亚硝氮"=w236) -> (w237:T10)
                    n166 = Bundle By Name(cluster=w245, "亚硝氮跨度值"=w243, "亚硝氮零点标准液浓度"=w242, "亚硝氮跨度标准液浓度"=w241, "亚硝氮标准液标准浓度"=w240, "亚硝氮零点标准液偏差"=w235, "亚硝氮跨度标准液偏差"=w234, "亚硝氮标准液标准偏差"=w233) -> (w244:T11)
                    n167 = global write "总磷总氮断电保存全局变量.vi" "质控参数设置"(w244) -> ()
                  }
                  frame 7 {
                    n168 = global write "总磷总氮断电保存全局变量.vi" "硅酸盐自动测试量程配置"(w252) -> ()
                    n169 = Bundle By Name(cluster=w251, "硅酸盐"=w249) -> (w250:T10)
                    n170 = Bundle By Name(cluster=w258, "硅酸盐跨度值"=w256, "硅酸盐零点标准液浓度"=w255, "硅酸盐跨度标准液浓度"=w254, "硅酸盐标准液标准浓度"=w253, "硅酸盐零点标准液偏差"=w248, "硅酸盐跨度标准液偏差"=w247, "硅酸盐标准液标准偏差"=w246) -> (w257:T11)
                    n171 = global write "总磷总氮断电保存全局变量.vi" "质控参数设置"(w257) -> ()
                  }
                  frame 8 {
                    n172 = global write "总磷总氮断电保存全局变量.vi" "硫化物自动测试量程配置"(w265) -> ()
                    n173 = Bundle By Name(cluster=w264, "硫化物"=w262) -> (w263:T10)
                    n174 = Bundle By Name(cluster=w271, "硫化物跨度值"=w269, "硫化物零点标准液浓度"=w268, "硫化物跨度标准液浓度"=w267, "硫化物标准液标准浓度"=w266, "硫化物零点标准液偏差"=w261, "硫化物跨度标准液偏差"=w260, "硫化物标准液标准偏差"=w259) -> (w270:T11)
                    n175 = global write "总磷总氮断电保存全局变量.vi" "质控参数设置"(w270) -> ()
                  }
                  frame 22 {
                    n176 = global write "总磷总氮断电保存全局变量.vi" "COD自动测试量程配置"(w278) -> ()
                    n177 = global write "总磷总氮断电保存全局变量.vi" "CODcr消解时长"(w279) -> ()
                    n178 = Bundle By Name(cluster=w277, "COD"=w275) -> (w276:T10)
                    n179 = Bundle By Name(cluster=w285, "COD跨度值"=w283, "COD零点标准液浓度"=w282, "COD跨度标准液浓度"=w281, "COD标准液标准浓度"=w280, "COD零点标准液偏差"=w274, "COD跨度标准液偏差"=w273, "COD标准液标准偏差"=w272) -> (w284:T11)
                    n180 = global write "总磷总氮断电保存全局变量.vi" "质控参数设置"(w284) -> ()
                  }
                  frame 21 {
                    n181 = global write "总磷总氮断电保存全局变量.vi" "CODMn自动测试量程配置"(w292) -> ()
                    n182 = global write "总磷总氮断电保存全局变量.vi" "CODmn消解时长"(w293) -> ()
                    n183 = Bundle By Name(cluster=w291, "CODMn"=w289) -> (w290:T10)
                    n184 = Bundle By Name(cluster=w299, "CODMn跨度值"=w297, "CODMn零点标准液浓度"=w296, "CODMn跨度标准液浓度"=w295, "CODMn标准液标准浓度"=w294, "CODMn零点标准液偏差"=w288, "CODMn跨度标准液偏差"=w287, "CODMn标准液标准偏差"=w286) -> (w298:T11)
                    n185 = global write "总磷总氮断电保存全局变量.vi" "质控参数设置"(w298) -> ()
                  }
                  frame 50 {
                    n186 = global write "总磷总氮断电保存全局变量.vi" "氟化物自动测试量程配置"(w306) -> ()
                    n187 = Bundle By Name(cluster=w305, "氟化物"=w303) -> (w304:T10)
                    n188 = Bundle By Name(cluster=w312, "氟化物跨度值"=w310, "氟化物零点标准液浓度"=w309, "氟化物跨度标准液浓度"=w308, "氟化物标准液标准浓度"=w307, "氟化物零点标准液偏差"=w302, "氟化物跨度标准液偏差"=w301, "氟化物标准液标准偏差"=w300) -> (w311:T11)
                    n189 = global write "总磷总氮断电保存全局变量.vi" "质控参数设置"(w311) -> ()
                  }
                }
                n190 = global write "总磷总氮断电保存全局变量.vi" "低量程上限"(w141) -> ()
              }
              frame #1 {
                n191 = Get Date/Time In Seconds() -> (seconds since 1Jan1904=w315:timestamp)
                n192 = property on="参数下拉列表" class="Ring (严格)"() -> ("RingText.Text"=w313:string)  [unwired: 2 in, 2 out]
                n193 = Bundle By Name(cluster=T7 {"时间"=timestamp(0 s since 1904-01-01), "参数"="", "日志信息"="", "流程参数"=""} ("data in"), "时间"=w315, "参数"=w313, "日志信息"="参数变更") -> (w316:T7)
                n194 = call "总磷总氮操作日志.vi"("data in"=w316) -> ()  [unwired: 10 in, 1 out]
                n195 = call "仪器配置写入.vi"() -> ()  [unwired: 11 in, 1 out]
              }
            }
          }
        }
      }
      event "通讯连接": Value Change {
        n196 = event-data() -> ("NewVal"=w318:bool)  [unwired: 1 in, 5 out]
        n197 = Flush Queue(queue=w319) -> (queue out=w320:refnum<queue>)  [unwired: 1 in, 2 out]
        n198 = case shown="假" w318 {
          tunnel: w320 -> [w321 w323]
          frame False {
            n199 = Enqueue Element At Opposite End(queue=w321, element=cluster{"命令":string, "data":variant} {"命令"="停用模块", "data"=variant} ("元素")) -> ()  [unwired: 2 in, 3 out]
          }
          frame True {
            n200 = Enqueue Element At Opposite End(queue=w323, element=cluster{"命令":string, "data":variant} {"命令"="启用模块", "data"=variant} ("元素")) -> ()  [unwired: 2 in, 3 out]
          }
        }
      }
    }
  }
  n201 = while {
    tunnel: w2 -> [w335]
    tunnel: w3 -> [w334]
    tunnel: w4 -> [w333]
    tunnel: w1 -> [w332]
    stop <- FALSE stop-if-true
    n202 = Wait on Occurrence(2:w332) -> (0:w326:bool)  [unwired: 2 in]
    n203 = flat-sequence {
      tunnel: w335 -> [w342]
      tunnel: w334 -> [w341]
      tunnel: w333 -> [w340]
      tunnel: [w339] -> w329
      tunnel: [w338] -> w328
      tunnel: [w337] -> w327
      tunnel: w326 -> [_]
      frame #0 {
        n204 = property class="Enum (严格)"(reference=w341) -> ("Value"=w338:enum16{"低量程", "高量程"})  [unwired: 1 in, 2 out]
        n205 = property class="Ring (严格)"(reference=w342) -> ("Value"=w339:u16)  [unwired: 1 in, 2 out]
        n206 = property class="Enum (严格)"(reference=w340) -> ("Value"=w337:T1)  [unwired: 1 in, 2 out]
      }
    }
    n207 = flat-sequence {
      tunnel: [w345] -> w331
      tunnel: [w344] -> w330
      tunnel: w329 -> [w343]
      tunnel: w328 -> [w345]
      tunnel: w327 -> [w344]
      tunnel: [w343] -> w325
      tunnel: w331 -> [w364]
      tunnel: w330 -> [w365]
      tunnel: w325 -> [w363]
      frame #0 {
      }
      frame #1 {
        n208 = call "量程参数读取.vi"("测量参数"=w363) -> ("error out"=w354:errorcluster, "量程参数读取"=w362:T6)  [unwired: 9 in]
        n209 = Unbundle By Name(w362) -> ("测量精度"=→"测量精度":u16, "检出限"=→"检出限":dbl, "上限"=→"高量程上限":dbl, "下限"=→"量程下限":dbl, "阈值（低->高）"=→"阈值（低->高）":dbl, "阈值（高->低）"=→"阈值（高->低）":dbl, "稀释度"=→"稀释度":dbl)
        n210 = call "公式读取.vi"("error in (no error)"=w354, "量程"=w364, "测量模式"=w365, "测量参数"=w363) -> ("error out"=w348:errorcluster, "公式"=w353:cluster{"X^2":dbl, "X":dbl, "b":dbl})  [unwired: 6 in]
        n211 = Unbundle By Name(w353) -> ("X^2"=→"二次多项式系数":dbl, "X"=→"曲线斜率":dbl, "b"=→"曲线截距":dbl)
        n212 = global read "VAR总磷总氮全局变量.vi" "MB session in"() -> (w347:refnum<class "MB_Master.lvclass">)
        n213 = case shown="1, 2, 21, 22" w363 {
          tunnel: [_ w368] -> w349
          tunnel: [w366 w374] -> _
          tunnel: w348 -> [w366 w369]
          tunnel: w347 -> [_ w372]
          tunnel: [_ w373] -> w346
          frame 0, Default {
          }
          frame 1, 2, 21, 22 {
            n214 = call "版本判断.vi"() -> ("仪器版本"=w371:T12)  [unwired: 11 in]
            n215 = case shown="\"A版\", 默认" w371 {
              tunnel: [w380 w384 w390] -> w370
              tunnel: w372 -> [w379 w385 w391]
              tunnel: [w376 w382 w388] -> w368
              tunnel: w369 -> [w378 _ w387]
              tunnel: [w375 w381 w386] -> w367
              frame "A版", Default {
                n216 = call "读取外设配置.vi"("error in (no error)"=w378, "MB session in"=w379) -> ("error out"=w380:errorcluster, "外设配置"=w377:T8, "MB session out"=w375:refnum<class "MB_Master.lvclass">)  [unwired: 7 in]
                n217 = Unbundle By Name(w377) -> ("消解温度下限"=w376:sgl)
              }
              frame "B版" {
                n218 = call "读取B版外设配置.vi"("MB session in"=w385) -> ("error out"=w384:errorcluster, "外设配置"=w383:T13, "MB session out"=w381:refnum<class "MB_Master.lvclass">)  [unwired: 8 in]
                n219 = Unbundle By Name(w383) -> ("消解温度下限"=w382:sgl)
              }
              frame "A1版" {
                n220 = call "读取A1外设配置.vi"("error in (no error)"=w387, "MB session in"=w391) -> ("error out"=w390:errorcluster, "外设配置"=w389:T14, "MB session out"=w386:refnum<class "MB_Master.lvclass">)  [unwired: 7 in]
                n221 = Unbundle By Name(w389) -> ("消解温度下限"=w388:sgl)
              }
            }
            n222 = call "盐度补偿值读取.vi"("Error in"=w370, "MB session in"=w367) -> ("error out"=w374:errorcluster, "盐度补偿值"=w373:sgl)  [unwired: 7 in, 1 out]
          }
        }
        "消解温度" <- w349
        "盐度补偿值" <- w346
      }
      frame #2 {
        n223 = Format Date/Time String() -> (date/time string=→"数据刷新时间":string)  [unwired: 3 in]
      }
    }
  }
  n224 = while {
    tunnel: w2 -> [w403]
    stop <- FALSE stop-if-true
    n225 = global read "总磷总氮断电保存全局变量.vi" "盐度自动补偿："() -> (w418:bool)
    n226 = property class="Ring (严格)"(reference=w403) -> ("Value"=w402:u16)  [unwired: 1 in, 2 out]
    n227 = global read "总磷总氮断电保存全局变量.vi" "跨度核查自动补测"() -> (w393:bool)
    n228 = global read "总磷总氮断电保存全局变量.vi" "MB通信方式选择"() -> (w417:enum16{"串口", "TCP"})
    n229 = global read "总磷总氮断电保存全局变量.vi" "VISA Resource"() -> (w422:refnum<visa-resource-name>)
    n230 = global read "总磷总氮断电保存全局变量.vi" "简易流程路径"() -> (w401:path)
    n231 = global read "总磷总氮断电保存全局变量.vi" "零点核查自动补测"() -> (w395:bool)
    n232 = global read "总磷总氮断电保存全局变量.vi" "标样核查自动补测"() -> (w394:bool)
    n233 = global read "总磷总氮断电保存全局变量.vi" "流程路径"() -> (w419:path)
    n234 = global read "总磷总氮断电保存全局变量.vi" "PORT"() -> (w421:string)
    n235 = local write "盐度自动补偿："(w418) -> ()
    n236 = global read "总磷总氮断电保存全局变量.vi" "质控参数设置"() -> (w412:T11)
    n237 = global read "总磷总氮断电保存全局变量.vi" "低量程上限"() -> (w400:T10)
    n238 = local write "跨度核查自动补测"(w393) -> ()
    n239 = local write "通信方式选择"(w417) -> ()
    n240 = local write "请选择串口:"(w422) -> ()
    n241 = local write "简易流程路径"(w401) -> ()
    n242 = local write "零点核查自动补测"(w395) -> ()
    n243 = local write "标样核查自动补测"(w394) -> ()
    n244 = local write "测试流程路径"(w419) -> ()
    n245 = local write "PORT"(w421) -> ()
    n246 = case shown="21" w402 {
      tunnel: [_ w437 w449 w460 w471 w482 w493 w504 w515 w527 w538 w550] -> w410
      tunnel: [_ w436 w448 _ _ _ _ _ _ w526 _ w539] -> w411
      tunnel: w412 -> [_ w435 w447 w459 w470 w481 w492 w503 w514 w525 w537 w549]
      tunnel: [_ w434 w446 w458 w469 w480 w491 w502 w513 w524 w536 w548] -> w413
      tunnel: [_ w433 w445 w457 w468 w479 w490 w501 w512 w523 w535 w547] -> w414
      tunnel: [_ w432 w444 w456 w467 w478 w489 w500 w511 w522 w534 w546] -> w415
      tunnel: [_ w431 w443 w455 w466 w477 w488 w499 w510 w521 w533 w545] -> w416
      tunnel: w400 -> [_ w430 w442 w454 w465 w476 w487 w498 w509 w520 w532 w544]
      tunnel: [0.0 ("COD") w429 w441 w453 w464 w475 w486 w497 w508 w519 w531 w543] -> w399
      tunnel: [_ w428 w440 w452 w463 w474 w485 w496 w507 w518 w530 w542] -> w398
      tunnel: [_ w427 w439 w451 w462 w473 w484 w495 w506 w517 w529 w541] -> w397
      tunnel: [_ w426 w438 w450 w461 w472 w483 w494 w505 w516 w528 w540] -> w396
      frame Default {
      }
      frame 1 {
        n247 = Unbundle By Name(w435) -> ("总磷跨度值"=w434:dbl, "总磷零点标准液浓度"=w433:dbl, "总磷跨度标准液浓度"=w432:dbl, "总磷标准液标准浓度"=w431:dbl, "总磷零点标准液偏差"=w428:dbl, "总磷跨度标准液偏差"=w427:dbl, "总磷标准液标准偏差"=w426:dbl)
        n248 = Unbundle By Name(w430) -> ("总磷"=w429:dbl)
        n249 = global read "总磷总氮断电保存全局变量.vi" "总磷消解时长"() -> (w436:dbl)
        n250 = global read "总磷总氮断电保存全局变量.vi" "总磷自动测试量程配置"() -> (w437:T15)
      }
      frame 2 {
        n251 = Unbundle By Name(w447) -> ("总氮跨度值"=w446:dbl, "总氮零点标准液浓度"=w445:dbl, "总氮跨度标准液浓度"=w444:dbl, "总氮标准液标准浓度"=w443:dbl, "总氮零点标准液偏差"=w440:dbl, "总氮跨度标准液偏差"=w439:dbl, "总氮标准液标准偏差"=w438:dbl)
        n252 = Unbundle By Name(w442) -> ("总氮"=w441:dbl)
        n253 = global read "总磷总氮断电保存全局变量.vi" "总氮消解时长"() -> (w448:dbl)
        n254 = global read "总磷总氮断电保存全局变量.vi" "总氮自动测试量程配置"() -> (w449:T15)
      }
      frame 3 {
        n255 = Unbundle By Name(w459) -> ("氨氮跨度值"=w458:dbl, "氨氮零点标准液浓度"=w457:dbl, "氨氮跨度标准液浓度"=w456:dbl, "氨氮标准液标准浓度"=w455:dbl, "氨氮零点标准液偏差"=w452:dbl, "氨氮跨度标准液偏差"=w451:dbl, "氨氮标准液标准偏差"=w450:dbl)
        n256 = Unbundle By Name(w454) -> ("氨氮"=w453:dbl)
        n257 = global read "总磷总氮断电保存全局变量.vi" "氨氮自动测试量程配置"() -> (w460:T15)
      }
      frame 4 {
        n258 = Unbundle By Name(w470) -> ("磷酸盐跨度值"=w469:dbl, "磷酸盐零点标准液浓度"=w468:dbl, "磷酸盐跨度标准液浓度"=w467:dbl, "磷酸盐标准液标准浓度"=w466:dbl, "磷酸盐零点标准液偏差"=w463:dbl, "磷酸盐跨度标准液偏差"=w462:dbl, "磷酸盐标准液标准偏差"=w461:dbl)
        n259 = Unbundle By Name(w465) -> ("磷酸盐"=w464:dbl)
        n260 = global read "总磷总氮断电保存全局变量.vi" "磷酸盐自动测试量程配置"() -> (w471:T15)
      }
      frame 5 {
        n261 = Unbundle By Name(w481) -> ("硝氮跨度值"=w480:dbl, "硝氮零点标准液浓度"=w479:dbl, "硝氮跨度标准液浓度"=w478:dbl, "硝氮标准液标准浓度"=w477:dbl, "硝氮零点标准液偏差"=w474:dbl, "硝氮跨度标准液偏差"=w473:dbl, "硝氮标准液标准偏差"=w472:dbl)
        n262 = Unbundle By Name(w476) -> ("硝氮"=w475:dbl)
        n263 = global read "总磷总氮断电保存全局变量.vi" "硝氮自动测试量程配置"() -> (w482:T15)
      }
      frame 6 {
        n264 = Unbundle By Name(w492) -> ("亚硝氮跨度值"=w491:dbl, "亚硝氮零点标准液浓度"=w490:dbl, "亚硝氮跨度标准液浓度"=w489:dbl, "亚硝氮标准液标准浓度"=w488:dbl, "亚硝氮零点标准液偏差"=w485:dbl, "亚硝氮跨度标准液偏差"=w484:dbl, "亚硝氮标准液标准偏差"=w483:dbl)
        n265 = Unbundle By Name(w487) -> ("亚硝氮"=w486:dbl)
        n266 = global read "总磷总氮断电保存全局变量.vi" "亚硝氮自动测试量程配置"() -> (w493:T15)
      }
      frame 7 {
        n267 = Unbundle By Name(w503) -> ("硅酸盐跨度值"=w502:dbl, "硅酸盐零点标准液浓度"=w501:dbl, "硅酸盐跨度标准液浓度"=w500:dbl, "硅酸盐标准液标准浓度"=w499:dbl, "硅酸盐零点标准液偏差"=w496:dbl, "硅酸盐跨度标准液偏差"=w495:dbl, "硅酸盐标准液标准偏差"=w494:dbl)
        n268 = Unbundle By Name(w498) -> ("硅酸盐"=w497:dbl)
        n269 = global read "总磷总氮断电保存全局变量.vi" "硅酸盐自动测试量程配置"() -> (w504:T15)
      }
      frame 8 {
        n270 = Unbundle By Name(w514) -> ("硫化物跨度值"=w513:dbl, "硫化物零点标准液浓度"=w512:dbl, "硫化物跨度标准液浓度"=w511:dbl, "硫化物标准液标准浓度"=w510:dbl, "硫化物零点标准液偏差"=w507:dbl, "硫化物跨度标准液偏差"=w506:dbl, "硫化物标准液标准偏差"=w505:dbl)
        n271 = Unbundle By Name(w509) -> ("硫化物"=w508:dbl)
        n272 = global read "总磷总氮断电保存全局变量.vi" "硫化物自动测试量程配置"() -> (w515:T15)
      }
      frame 22 {
        n273 = Unbundle By Name(w525) -> ("COD跨度值"=w524:dbl, "COD零点标准液浓度"=w523:dbl, "COD跨度标准液浓度"=w522:dbl, "COD标准液标准浓度"=w521:dbl, "COD零点标准液偏差"=w518:dbl, "COD跨度标准液偏差"=w517:dbl, "COD标准液标准偏差"=w516:dbl)
        n274 = Unbundle By Name(w520) -> ("COD"=w519:dbl)
        n275 = global read "总磷总氮断电保存全局变量.vi" "CODcr消解时长"() -> (w526:dbl)
        n276 = global read "总磷总氮断电保存全局变量.vi" "COD自动测试量程配置"() -> (w527:T15)
      }
      frame 50 {
        n277 = Unbundle By Name(w537) -> ("氟化物跨度值"=w536:dbl, "氟化物零点标准液浓度"=w535:dbl, "氟化物跨度标准液浓度"=w534:dbl, "氟化物标准液标准浓度"=w533:dbl, "氟化物零点标准液偏差"=w530:dbl, "氟化物跨度标准液偏差"=w529:dbl, "氟化物标准液标准偏差"=w528:dbl)
        n278 = Unbundle By Name(w532) -> ("氟化物"=w531:dbl)
        n279 = global read "总磷总氮断电保存全局变量.vi" "氟化物自动测试量程配置"() -> (w538:T15)
      }
      frame 21 {
        n280 = Unbundle By Name(w549) -> ("CODMn跨度值"=w548:dbl, "CODMn零点标准液浓度"=w547:dbl, "CODMn跨度标准液浓度"=w546:dbl, "CODMn标准液标准浓度"=w545:dbl, "CODMn零点标准液偏差"=w542:dbl, "CODMn跨度标准液偏差"=w541:dbl, "CODMn标准液标准偏差"=w540:dbl)
        n281 = Unbundle By Name(w544) -> ("CODMn"=w543:dbl)
        n282 = global read "总磷总氮断电保存全局变量.vi" "CODMn自动测试量程配置"() -> (w550:T15)
        n283 = global read "总磷总氮断电保存全局变量.vi" "CODcr消解时长"() -> (w539:dbl)
      }
    }
    "消解时长" <- w411
    "低量程上限" <- w399
    n284 = global read "总磷总氮断电保存全局变量.vi" "IP"() -> (w420:string)
    n285 = local write "IP"(w420) -> ()
    n286 = Wait (ms)(milliseconds to wait=u32 1000 ("等待时间（毫秒）")) -> ()  [unwired: 1 out]
    n287 = local write "跨度值"(w413) -> ()
    n288 = local write "零点核查标液浓度"(w414) -> ()
    n289 = local write "跨度核查标液浓度"(w415) -> ()
    n290 = local write "标样核查标液浓度"(w416) -> ()
    n291 = local write "零点核查标液偏差"(w398) -> ()
    n292 = local write "跨度核查标液偏差"(w397) -> ()
    n293 = local write "标样核查标液偏差"(w396) -> ()
    n294 = To Unsigned Word Integer(number=w410) -> (unsigned 16bit integer=w409:T16)
    n295 = Unbundle By Name(w409) -> ("水样测试量程模式"=w408:u16, "空白核查量程模式"=w406:u16, "跨度核查量程模式"=w405:u16, "加标回收量程模式"=w404:u16, "标样核查量程模式"=w407:u16)
    n296 = local write "水样测试量程模式"(w408) -> ()
    n297 = local write "零点核查量程模式"(w406) -> ()
    n298 = local write "跨度核查量程模式"(w405) -> ()
    n299 = local write "加标回收量程模式"(w404) -> ()
    n300 = local write "标样核查量程模式"(w407) -> ()
  }
